vi "Wait For Command.vi"(8 "error in (no error)":errorcluster, 9 "timeout in ms (0)":i32 format="%d ms", 11 "Plugin Thread in":refnum<class "Plugin Thread.lvclass">) -> (0 "error out":errorcluster, 2 "command":T1={"Command"=enum."Start", "Parameters"={"arg1"=0, "arg2"=0}}, 3 "Plugin Thread out":refnum<class "Plugin Thread.lvclass">)   [LabVIEW 2020, in "DSF Core.lvlib" / "Plugin Thread.lvclass"]
uses:
  Plugin Thread.lvclass
  Thread.lvclass
  Commands.ctl
  Interface/Plugin/Command Parameters.ctl
  Interface/Plugin/Plugin Interface.lvclass
  Command Data.ctl
  Interface/Plugin/Response.ctl
  C:/Users/nitest/Desktop/Git/niveristand-data-sharing-framework-custom-device/Source/Core/Classes/Thread/Thread.lvclass
  C:/Users/nitest/Desktop/Git/niveristand-data-sharing-framework-custom-device/Source/Core/Classes/Thread/Plugin/Plugin Thread.lvclass
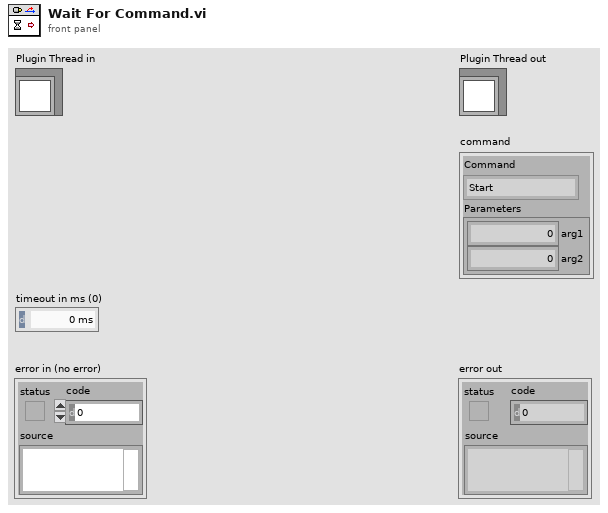
[diagram p1: front panel]
types:
  T1 = typedef "DSF Core.lvlib/Plugin Thread.lvclass/Command Data.ctl" = cluster{"Command":T2, "Parameters":T3}
  T2 = typedef "DSF Core.lvlib/Plugin Thread.lvclass/Commands.ctl" = enum8{"Idle", "Error", "Start", "Rx", "Tx", "Shutdown"}
  T3 = typedef "DSF Core.lvlib/Plugin Interface.lvclass/Command Parameters.ctl" = cluster{"arg1":u64, "arg2":u64}
  T4 = typedef "DSF Core.lvlib/Plugin Interface.lvclass/Command Data.ctl" = cluster{"Command":T5, "Parameters":T3}
  T5 = typedef "DSF Core.lvlib/Plugin Interface.lvclass/Command.ctl" = enum8{"Idle", "Start", "Set Inline Buffer", "Rx", "Tx", "Shutdown", "Error"}
  T6 = typedef "DSF Core.lvlib/Plugin Interface.lvclass/Response.ctl" = enum8{"General Ack", "Shutting Down"}
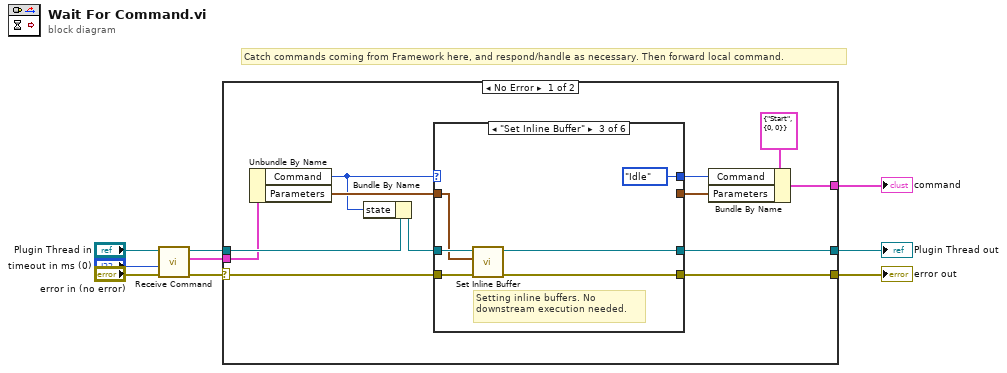
[diagram p0: block diagram]
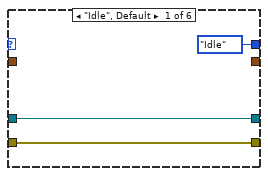
[diagram p2: hidden frame]
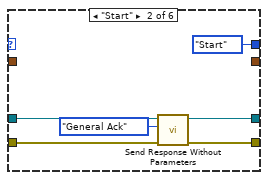
[diagram p3: hidden frame]
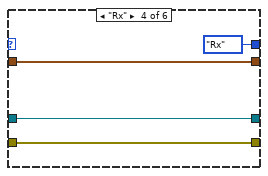
[diagram p4: hidden frame]
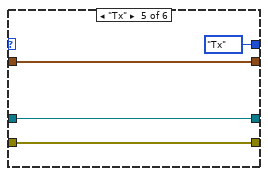
[diagram p5: hidden frame]
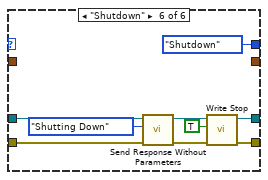
[diagram p6: hidden frame]
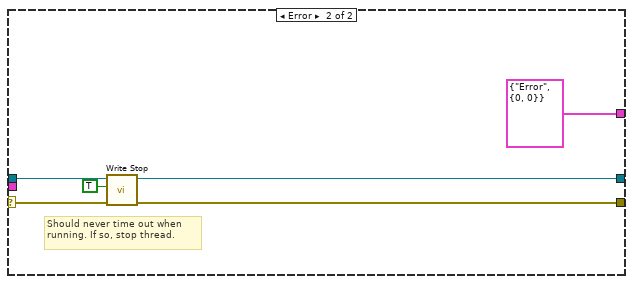
[diagram p7: hidden frame]
diagram:
  # "Catch commands coming from Framework here, and respond/handle as necessary. Then forward local command."
  n1 = call "Receive Command.vi"("error in (no error)"="error in (no error)", "timeout in ms (0)"="timeout in ms (0)", "Plugin Thread in"="Plugin Thread in") -> ("error out"=w6:errorcluster, "command"=w2:T4, "Plugin Thread out"=w4:refnum<class "Plugin Thread.lvclass">)  [unwired: 6 in]
  n2 = case shown="No Error" w6 {
    selector: w6 -> [w20 w58]
    tunnel: [w18 w57] -> w5
    tunnel: w4 -> [w14 w56]
    tunnel: [w19 w55] -> w3
    tunnel: w2 -> [w11 _]
    tunnel: [w16 T1 {"Command"=enum."Error", "Parameters"={"arg1"=0, "arg2"=0}} ("Command")] -> w1
    frame No Error {
      n3 = Unbundle By Name(w11) -> ("Command"=w10:T5, "Parameters"=w13:T3)
      n4 = Bundle By Name(cluster=w14, "state"=w10) -> (w21:refnum<class "Plugin Thread.lvclass">)
      n5 = case shown="\"Set Inline Buffer\"" w10 {
        tunnel: w21 -> [w24 w29 w35 w39 w43 w50]
        tunnel: w20 -> [w23 w26 w34 w38 w42 w49]
        tunnel: [w24 w28 w32 w39 w43 w47] -> w19
        tunnel: [w23 w27 w33 w38 w42 w45] -> w18
        tunnel: [Commands."Idle" ("command") Commands."Start" ("command") Commands."Idle" ("command") Commands."Rx" ("command") Commands."Tx" ("command") Commands."Shutdown" ("command")] -> w15
        tunnel: w13 -> [_ _ w31 w40 w44 _]
        tunnel: [_ _ _ w40 w44 _] -> w12
        frame "Idle", Default {
        }
        frame "Start" {
          n6 = call "Send Response Without Parameters.vi"("error in (no error)"=w26, "response"=Response."General Ack", "Plugin Thread in"=w29) -> ("error out"=w27:errorcluster, "Plugin Thread out"=w28:refnum<class "Plugin Thread.lvclass">)  [unwired: 7 in]
        }
        frame "Set Inline Buffer" {
          # "Setting inline buffers. No downstream execution needed."
          n7 = call "Set Inline Buffer.vi"("error in (no error)"=w34, "command parameters"=w31, "Plugin Thread in"=w35) -> ("error out"=w33:errorcluster, "Plugin Thread out"=w32:refnum<class "Plugin Thread.lvclass">)  [unwired: 7 in]
        }
        frame "Rx" {
        }
        frame "Tx" {
        }
        frame "Shutdown" {
          n8 = call "Send Response Without Parameters.vi"("error in (no error)"=w49, "response"=Response."Shutting Down", "Plugin Thread in"=w50) -> ("error out"=w46:errorcluster, "Plugin Thread out"=w48:refnum<class "Plugin Thread.lvclass">)  [unwired: 7 in]
          n9 = call "Write Stop.vi"("error in (no error)"=w46, "stop"=TRUE, "Thread in"=w48) -> ("error out"=w45:errorcluster, "Thread out"=w47:refnum<class "Plugin Thread.lvclass">)  [unwired: 7 in]
        }
      }
      n10 = Bundle By Name(cluster=T1 {"Command"=enum."Start", "Parameters"={"arg1"=0, "arg2"=0}} ("Command"), "Command"=w15, "Parameters"=w12) -> (w16:T1)
    }
    frame Error {
      # "Should never time out when running. If so, stop thread."
      n11 = call "Write Stop.vi"("error in (no error)"=w58, "stop"=TRUE, "Thread in"=w56) -> ("error out"=w57:errorcluster, "Thread out"=w55:refnum<class "Plugin Thread.lvclass">)  [unwired: 7 in]
    }
  }
  "error out" <- w5
  "Plugin Thread out" <- w3
  "command" <- w1
